vi "EtherCAT Write by Node U8Array.vi"(6 "data":u8[](array[numeric]), 8 "error in (no error)":errorcluster, 9 "startAddr":u16, 10 "nodeAddr":u16, 11 "masterHdl in":T1) -> (0 "error out":errorcluster, 3 "masterHdl out":T1)   [LabVIEW 2017, in "NI_Robotics_KUKA youBot Host.lvlib"]
uses:
  <vilib>/robotics/KUKA youBot/NI_Robotics_KUKA youBot Host.lvlib
  <vilib>/robotics/KUKA youBot/EtherCAT/LowLevel/Mater Handler.ctl
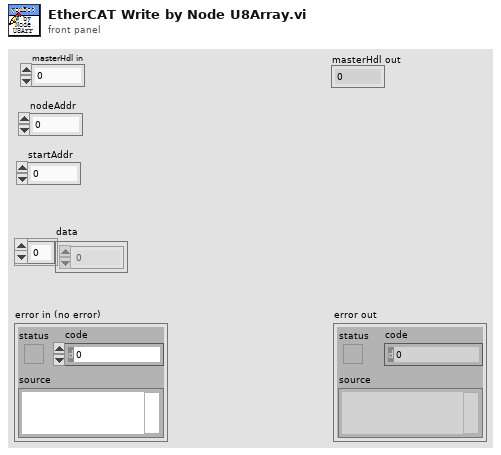
[diagram p1: front panel]
types:
  T1 = typedef "NI_Robotics_KUKA youBot Host.lvlib/Mater Handler.ctl" = i32
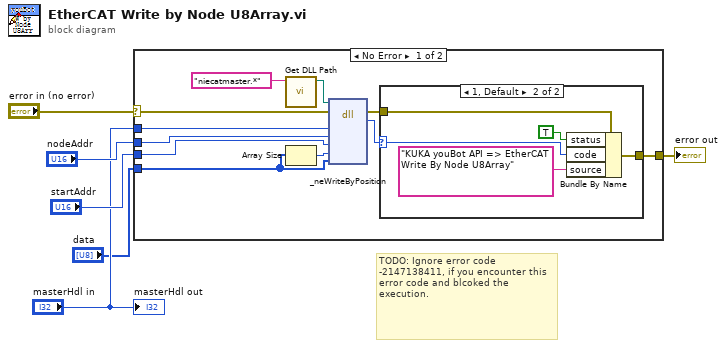
[diagram p0: block diagram]
diagram:
  # "TODO: Ignore error code -2147138411, if you encounter this error code and blcoked the execution."
  n1 = case shown="No Error" "error in (no error)" {
    selector: "error in (no error)" -> [w15 w24]
    tunnel: "data" -> [w10 _]
    tunnel: "startAddr" -> [w17 _]
    tunnel: "nodeAddr" -> [w16 _]
    tunnel: "masterHdl in" -> [w11 _]
    tunnel: [w12 w24] -> w3
    frame No Error {
      n2 = call <vilib>:"Get DLL Path.vi"("dll name"="niecatmaster.*") -> ("Path"=w7:path)  [unwired: 10 in]
      n3 = Array Size(array=w10) -> (size(s)=w9:i32)
      n4 = dll-call lib="C:/Program Files (x86)/National Instruments/LabVIEW 2012/resource/Framework/Providers/niecatmaster.*" fn="_neWriteByPosition"(path in=w7, error in=w15, "masterRef"=w11, "posAddr"=w16, "startAddr"=w17, "dataLen"=w9, "data"=w10) -> (error out=w13:errorcluster, "error"=w14:i32)  [unwired: 6 in, 1 out]
      n5 = case shown="1, Default" w14 {
        selector: w14 -> [_ w21]
        tunnel: w13 -> [w18 w23]
        tunnel: [w18 w20] -> w12
        frame 0 {
        }
        frame 1, Default {
          n6 = Bundle By Name(cluster=w23, "status"=TRUE, "code"=w21, "source"="KUKA youBot API => EtherCAT Write By Node U8Array") -> (w20:errorcluster)
        }
      }
    }
    frame Error {
    }
  }
  "error out" <- w3
  "masterHdl out" <- "masterHdl in"
